vi "json_load.vi"(8 "error in (no error)":errorcluster, 11 "json":string) -> (0 "error out":errorcluster, 3 "elements":T1[](array[typedef]))   [LabVIEW 2017]
uses:
  json_element.ctl
  json_element_type.ctl
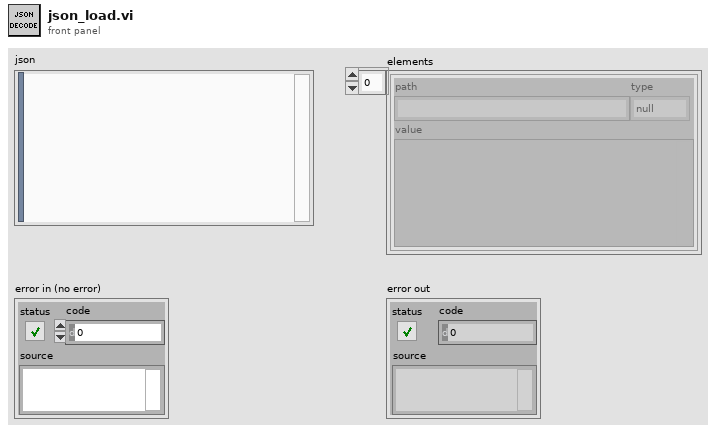
[diagram p1: front panel]
types:
  T1 = typedef "json_element.ctl" = cluster{"path":string, "type":T2, "value":variant}
  T2 = typedef "json_element_type.ctl" = enum8{"null", "bool", "int", "uint", "float", "string", "array", "object"}
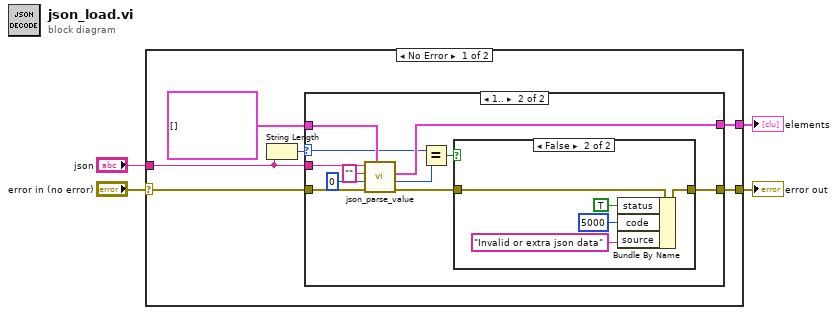
[diagram p0: block diagram]
diagram:
  n1 = case shown="No Error" "error in (no error)" {
    selector: "error in (no error)" -> [w10 w30]
    tunnel: "json" -> [w7 _]
    tunnel: [w9 _] -> w1
    tunnel: [w8 w30] -> w2
    frame No Error {
      n2 = String Length(string=w7) -> (length=w5:i32)
      n3 = case shown="1.." w5 {
        selector: w5 -> [_ w13]
        tunnel: w10 -> [w11 w23]
        tunnel: [w12 w22] -> w9
        tunnel: [w11 w21] -> w8
        tunnel: w7 -> [_ w20]
        tunnel: T1[] [] ("elements in") -> [w12 w14]
        frame ..0 {
        }
        frame 1.. {
          n4 = call "json_parse_value.vi"("elements in"=w14, "error in (no error)"=w23, "offset (0)"=0, "path"="" ("key"), "data"=w20) -> ("error out"=w19:errorcluster, "offset past match"=w17:i32, "elements out"=w22:T1[])  [unwired: 4 in]
          n5 = Equal?(x=w13, y=w17) -> (x = y?=w16:bool)
          n6 = case shown="False" w16 {
            tunnel: w19 -> [w24 w29]
            tunnel: [w24 w28] -> w21
            frame True {
            }
            frame False {
              n7 = Bundle By Name(cluster=w29, "status"=TRUE, "code"=5000, "source"="Invalid or extra json data") -> (w28:errorcluster)
            }
          }
        }
      }
    }
    frame Error {
    }
  }
  "error out" <- w2
  "elements" <- w1
